vi "IntensityGraphOperation.vi"(2 "Op-Mode":T1(ring), 3 "Ref Array":dbl[](array[numeric]), 5 "Data Array":dbl[][](array[numeric])) -> (1 "Data Array out":dbl[][](array[numeric]))   [LabVIEW 2025]
doc: "Author: Scott Hannahs <sth@magnet.fsu.edu>\n\nThis software is licensed for use under the “MIT License\"\nCopyright (c) 2025 Scott Hannahs, sth@sth@magnet.sthnet.net\n\nPermission is hereby granted, free of charge, to any person obtaining a copy of this software and associated documentation files (the \"Software\"), to deal in the Software without restriction, including without limitation the rights to use, copy, modify, merge, publish, distribute, sublicense, and/or sell copies of the Software, and to permit persons to whom the Software is furnished to do so, subject to the following conditions: The above copyright notice and this permission notice shall be included in all copies or substantial portions of the Software.\n\nTHE SOFTWARE IS PROVIDED \"AS IS\", WITHOUT WARRANTY OF ANY KIND, EXPRESS OR IMPLIED, INCLUDING BUT NOT LIMITED TO THE WARRANTIES OF MERCHANTABILITY, FITNESS FOR A PARTICULAR PURPOSE AND NONINFRINGEMENT. IN NO EVENT SHALL THE AUTHORS OR COPYRIGHT HOLDERS BE LIABLE FOR ANY CLAIM, DAMAGES OR OTHER LIABILITY, WHETHER IN AN ACTION OF CONTRACT, TORT OR OTHERWISE, ARISING FROM, OUT OF OR IN CONNECTION WITH THE SOFTWARE OR THE USE OR OTHER DEALINGS IN THE SOFTWARE."
uses:
  <vilib>/Analysis/2dsp.llb/Power Spectrum (DBL).vi
  <vilib>/Analysis/NI_AALPro.lvlib
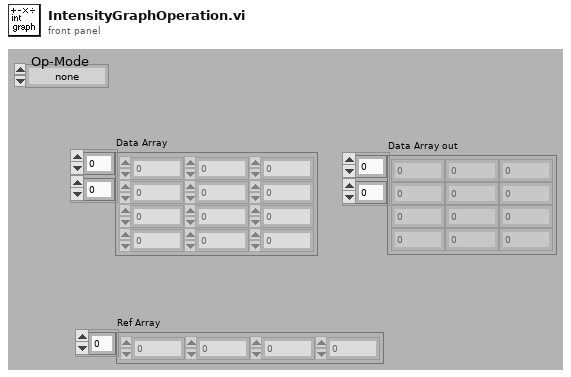
[diagram p1: front panel]
types:
  T1 = enum16{"none", " + ", " - ", " * ", " / ", "Integral", "Differential", "FFT"}
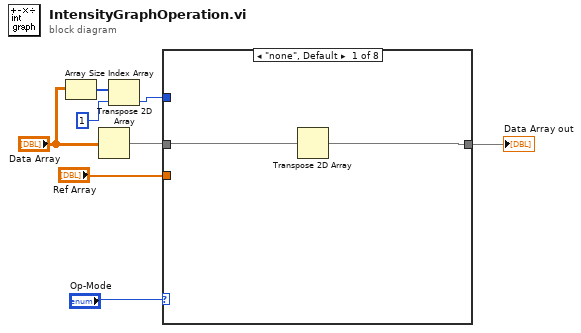
[diagram p0: block diagram]
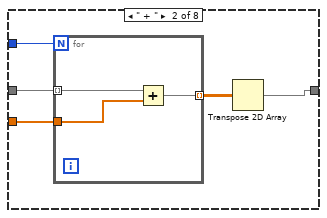
[diagram p2: hidden frame]
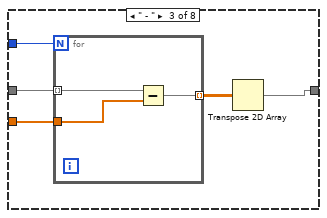
[diagram p3: hidden frame]
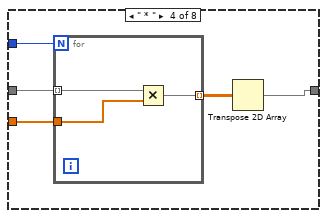
[diagram p4: hidden frame]
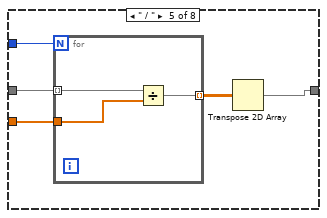
[diagram p5: hidden frame]
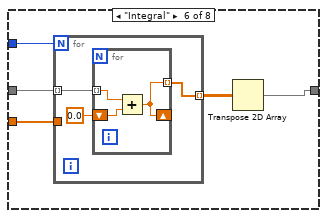
[diagram p6: hidden frame]
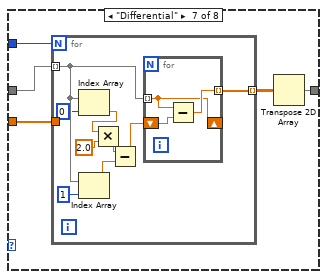
[diagram p7: hidden frame]
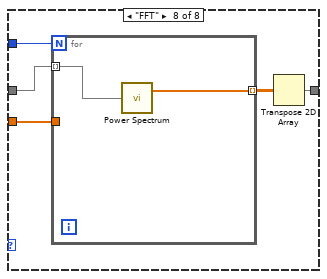
[diagram p8: hidden frame]
diagram:
  n1 = Array Size(array="Data Array") -> (size(s)=w6:i32[])
  n2 = Transpose 2D Array(2D array="Data Array") -> (transposed array=w2:dbl[][])
  n3 = Index Array(array=w6, index=1) -> (element=w4:i32)
  n4 = case shown="\"none\", Default" "Op-Mode" {
    tunnel: [w10 w11 w19 w27 w35 w43 w54 w71] -> w7
    tunnel: w2 -> [w9 w14 w22 w30 w38 w46 w57 w74]
    tunnel: w4 -> [_ w15 w23 w31 w39 w47 w58 w75]
    tunnel: "Ref Array" -> [_ w13 w21 w29 w37 w45 w56 w73]
    frame "none", Default {
      n5 = Transpose 2D Array(2D array=w9) -> (transposed array=w10:dbl[][])
    }
    frame " + " {
      n6 = for {
        N: w15 -> [_]
        tunnel: w14 -> [w16] mode=indexing
        tunnel: w13 -> [w18]
        tunnel: [w17] -> w12 mode=indexing
        n7 = Add(x=w16, y=w18) -> (x+y=w17:dbl[])
      }
      n8 = Transpose 2D Array(2D array=w12) -> (transposed array=w11:dbl[][])
    }
    frame " - " {
      n9 = for {
        N: w23 -> [_]
        tunnel: w22 -> [w24] mode=indexing
        tunnel: w21 -> [w26]
        tunnel: [w25] -> w20 mode=indexing
        n10 = Subtract(x=w24, y=w26) -> (x-y=w25:dbl[])
      }
      n11 = Transpose 2D Array(2D array=w20) -> (transposed array=w19:dbl[][])
    }
    frame " * " {
      n12 = for {
        N: w31 -> [_]
        tunnel: w30 -> [w32] mode=indexing
        tunnel: w29 -> [w34]
        tunnel: [w33] -> w28 mode=indexing
        n13 = Multiply(x=w32, y=w34) -> (x*y=w33:dbl[])
      }
      n14 = Transpose 2D Array(2D array=w28) -> (transposed array=w27:dbl[][])
    }
    frame " / " {
      n15 = for {
        N: w39 -> [_]
        tunnel: w38 -> [w40] mode=indexing
        tunnel: w37 -> [w42]
        tunnel: [w41] -> w36 mode=indexing
        n16 = Divide(x=w40, y=w42) -> (x/y=w41:dbl[])
      }
      n17 = Transpose 2D Array(2D array=w36) -> (transposed array=w35:dbl[][])
    }
    frame "Integral" {
      n18 = for {
        N: w47 -> [_]
        tunnel: w46 -> [w50] mode=indexing
        tunnel: w45 -> [_]
        tunnel: [w48] -> w44 mode=indexing
        n19 = for {
          tunnel: w50 -> [w52] mode=indexing
          shift-right: [w51] -> _
          shift-left: 0.0 ("Numeric") -> [w53]
          tunnel: [w51] -> w48 mode=indexing
          n20 = Add(x=w52, y=w53) -> (x+y=w51:dbl)
        }
      }
      n21 = Transpose 2D Array(2D array=w44) -> (transposed array=w43:dbl[][])
    }
    frame "Differential" {
      n22 = for {
        N: w58 -> [_]
        tunnel: w57 -> [w66] mode=indexing
        tunnel: w56 -> [_]
        tunnel: [w67] -> w55 mode=indexing
        n23 = Index Array(array=w66, index=0) -> (element=w63:dbl)
        n24 = Index Array(array=w66, index=1) -> (element=w61:dbl)
        n25 = Multiply(x=w63, y=2.0) -> (x*y=w60:dbl)
        n26 = Subtract(x=w60, y=w61) -> (x-y=w59:dbl)
        n27 = for {
          tunnel: w66 -> [w68] mode=indexing
          shift-right: [w68] -> _
          shift-left: w59 -> [w70]
          tunnel: [w69] -> w67 mode=indexing
          n28 = Subtract(x=w68, y=w70) -> (x-y=w69:dbl)
        }
      }
      n29 = Transpose 2D Array(2D array=w55) -> (transposed array=w54:dbl[][])
    }
    frame "FFT" {
      n30 = for {
        N: w75 -> [_]
        tunnel: w74 -> [w77] mode=indexing
        tunnel: w73 -> [_]
        tunnel: [w76] -> w72 mode=indexing
        n31 = call-poly <vilib>:"Power Spectrum.vi"("X"=w77) -> ("Power Spectrum"=w76:dbl[])  [unwired: 1 out]
      }
      n32 = Transpose 2D Array(2D array=w72) -> (transposed array=w71:dbl[][])
    }
  }
  "Data Array out" <- w7
